vi "calculate image sharpness.vi"(8 "error in (no error)":errorcluster, 9 "Sharpness measure":T1, 10 "Runtime cluster.Image array (floats)":dbl[][](array[numeric]), 11 "Autofocus in":refnum<class "Autofocus.lvclass">) -> (0 "error out":errorcluster, 2 "sharpness out":dbl, 3 "Autofocus out":refnum<class "Autofocus.lvclass">)   [LabVIEW 2012, in "Autofocus.lvclass"]
uses:
  Autofocus.lvclass
  Sharpness Measure.ctl
  Autofocus.lvclass/Autofocus.ctl
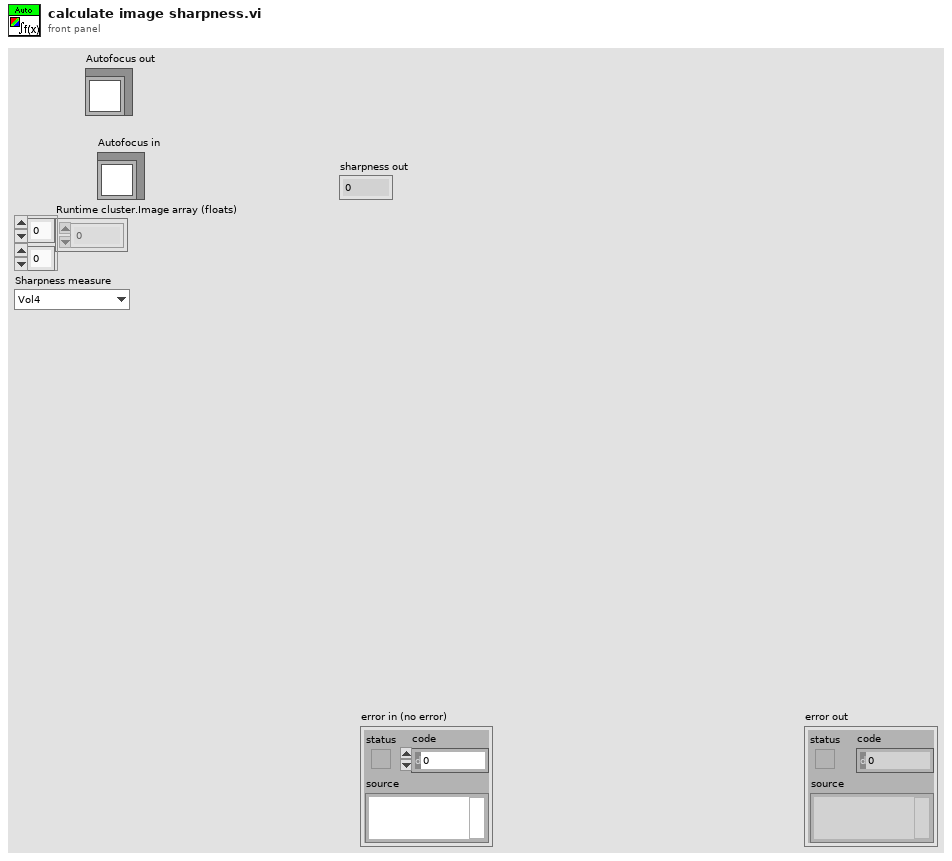
[diagram p1: front panel]
types:
  T1 = typedef "Autofocus.lvclass/Sharpness Measure.ctl" = enum16{"Vol4", "Gradient Square"}
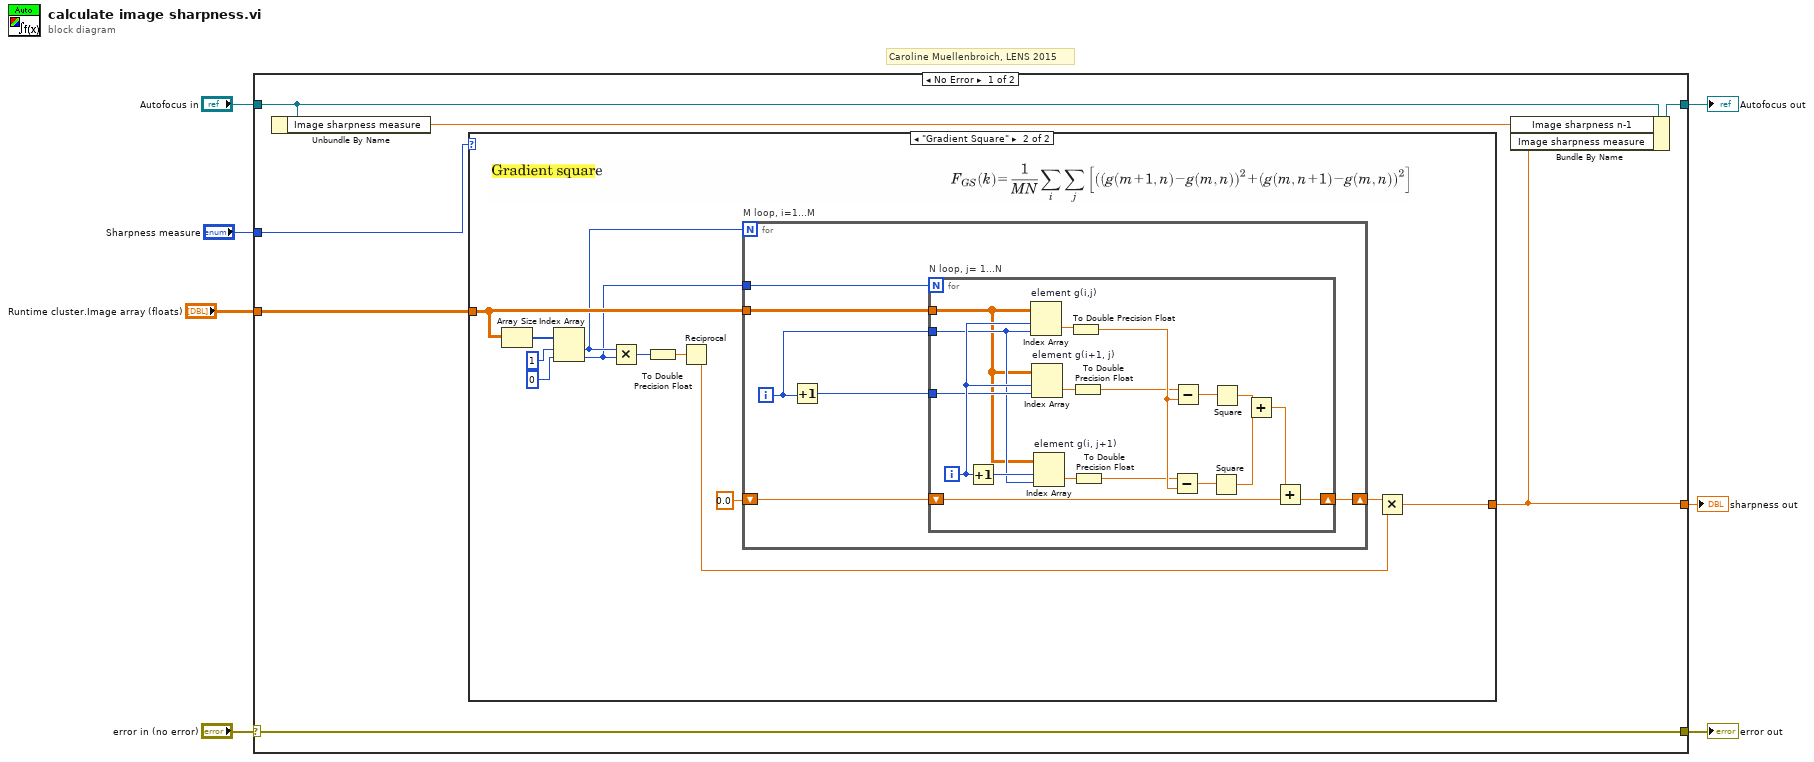
[diagram p0: block diagram]
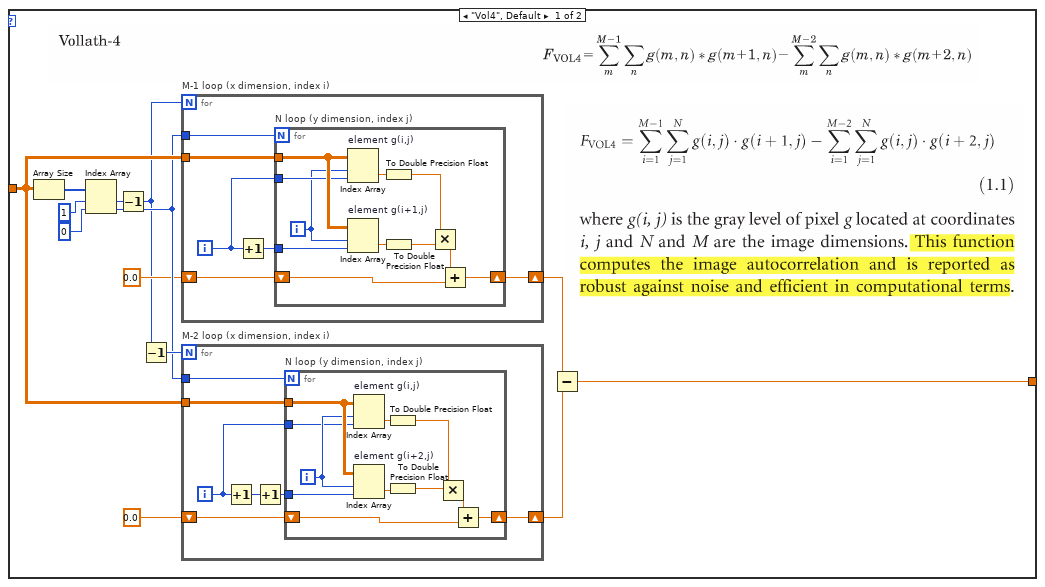
[diagram p2: hidden frame]
diagram:
  # "Caroline Muellenbroich, LENS 2015"
  n1 = case shown="No Error" "error in (no error)" {
    selector: "error in (no error)" -> [w14 w100]
    tunnel: [w14 w100] -> w6
    tunnel: [w12 w99] -> w4
    tunnel: "Autofocus in" -> [w13 w99]
    tunnel: [w10 _] -> w3
    tunnel: "Runtime cluster.Image array (floats)" -> [w9 _]
    tunnel: "Sharpness measure" -> [w8 _]
    frame No Error {
      n2 = Unbundle By Name(w13) -> ("Image sharpness measure"=w11:dbl)
      n3 = case shown="\"Gradient Square\"" w8 {
        tunnel: w9 -> [w22 w71]
        tunnel: [w16 w66] -> w10
        frame "Vol4", Default {
          n4 = Array Size(array=w22) -> (size(s)=w27:i32[])
          n5 = Index Array(array=w27, index #1=1 ("index"), index #2=0 ("index")) -> (element #1=w23:i32, element #2=w21:i32)
          n6 = Decrement(x=w23) -> (x-1=w15:i32)
          n7 = Decrement(x=w15) -> (x-1=w24:i32)
          n8 = for "M-1 loop (x dimension, index i)" {
            N: w15 -> [_]
            tunnel: w22 -> [w51]
            tunnel: w21 -> [w50]
            shift-right: [w47] -> w20
            shift-left: 0.0 -> [w46]
            i -> [w49]
            n9 = Increment(x=w49) -> (x+1=w48:i32)
            n10 = for "N loop (y dimension, index j)" {
              N: w50 -> [_]
              tunnel: w51 -> [w61]
              shift-right: [w54] -> w47
              shift-left: w46 -> [w62]
              tunnel: w49 -> [w59]
              tunnel: w48 -> [w57]
              i -> [w58]
              n11 = Index Array "element g(i,j)"(array=w61, index (row)=w58, index (col)=w59) -> (element=w56:dbl)
              n12 = Index Array "element g(i+1,j)"(array=w61, index (row)=w58, index (col)=w57) -> (element=w55:dbl)
              n13 = To Double Precision Float(number=w56) -> (double precision float=w52:dbl)
              n14 = To Double Precision Float(number=w55) -> (double precision float=w53:dbl)
              n15 = Multiply(x=w52, y=w53) -> (x*y=w60:dbl)
              n16 = Add(x=w60, y=w62) -> (x+y=w54:dbl)
            }
          }
          n17 = for "M-2 loop (x dimension, index i)" {
            N: w24 -> [_]
            tunnel: w22 -> [w33]
            tunnel: w21 -> [w34]
            shift-right: [w29] -> w19
            shift-left: 0.0 -> [w28]
            i -> [w32]
            n18 = Increment(x=w32) -> (x+1=w31:i32)
            n19 = Increment(x=w31) -> (x+1=w30:i32)
            n20 = for "N loop (y dimension, index j)" {
              N: w34 -> [_]
              tunnel: w33 -> [w42]
              tunnel: w32 -> [w40]
              tunnel: w30 -> [w39]
              shift-right: [w38] -> w29
              shift-left: w28 -> [w37]
              i -> [w41]
              n21 = Index Array "element g(i,j)"(array=w42, index (row)=w41, index (col)=w40) -> (element=w44:dbl)
              n22 = Index Array "element g(i+2,j)"(array=w42, index (row)=w41, index (col)=w39) -> (element=w45:dbl)
              n23 = To Double Precision Float(number=w44) -> (double precision float=w35:dbl)
              n24 = To Double Precision Float(number=w45) -> (double precision float=w36:dbl)
              n25 = Multiply(x=w35, y=w36) -> (x*y=w43:dbl)
              n26 = Add(x=w43, y=w37) -> (x+y=w38:dbl)
            }
          }
          n27 = Subtract(x=w20, y=w19) -> (x-y=w16:dbl)
        }
        frame "Gradient Square" {
          n28 = Array Size(array=w71) -> (size(s)=w74:i32[])
          n29 = Index Array(array=w74, index #1=1 ("index"), index #2=0 ("index")) -> (element #1=w64:i32, element #2=w63:i32)
          n30 = Multiply(x=w64, y=w63) -> (x*y=w70:i32)
          n31 = To Double Precision Float(number=w70) -> (double precision float=w69:dbl)
          n32 = Reciprocal(x=w69) -> (1/x=w65:dbl)
          n33 = for "M loop, i=1...M" {
            N: w64 -> [_]
            tunnel: w71 -> [w80]
            tunnel: w63 -> [w79]
            shift-right: [w76] -> w67
            shift-left: 0.0 -> [w75]
            i -> [w78]
            n34 = Increment(x=w78) -> (x+1=w77:i32)
            n35 = for "N loop, j= 1...N" {
              N: w79 -> [_]
              tunnel: w80 -> [w94]
              tunnel: w78 -> [w95]
              tunnel: w77 -> [w97]
              shift-right: [w84] -> w76
              shift-left: w75 -> [w86]
              i -> [w98]
              n36 = Increment(x=w98) -> (x+1=w96:i32)
              n37 = Index Array "element g(i,j)"(array=w94, index (row)=w98, index (col)=w95) -> (element=w89:dbl)
              n38 = Index Array "element g(i+1, j)"(array=w94, index (row)=w98, index (col)=w97) -> (element=w93:dbl)
              n39 = Index Array "element g(i, j+1)"(array=w94, index (row)=w96, index (col)=w95) -> (element=w90:dbl)
              n40 = To Double Precision Float(number=w89) -> (double precision float=w83:dbl)
              n41 = To Double Precision Float(number=w93) -> (double precision float=w82:dbl)
              n42 = To Double Precision Float(number=w90) -> (double precision float=w81:dbl)
              n43 = Subtract(x=w81, y=w83) -> (x-y=w91:dbl)
              n44 = Subtract(x=w82, y=w83) -> (x-y=w92:dbl)
              n45 = Square(x=w91) -> (x^2=w87:dbl)
              n46 = Square(x=w92) -> (x^2=w88:dbl)
              n47 = Add(x=w88, y=w87) -> (x+y=w85:dbl)
              n48 = Add(x=w85, y=w86) -> (x+y=w84:dbl)
            }
          }
          n49 = Multiply(x=w67, y=w65) -> (x*y=w66:dbl)
        }
      }
      n50 = Bundle By Name(cluster=w13, "Image sharpness n-1"=w11, "Image sharpness measure"=w10) -> (w12:refnum<class "Autofocus.lvclass">)
    }
    frame Error {
    }
  }
  "error out" <- w6
  "Autofocus out" <- w4
  "sharpness out" <- w3
